vi "Example Property Node 1.vi"() -> ()   [LabVIEW 2018]
panel:
  out "Connected Wire":refnum<vi>
  out "error out":errorcluster
  out "reference out":refnum<vi>
  in  "error in (no error)":errorcluster
  in  "reference":refnum<vi>
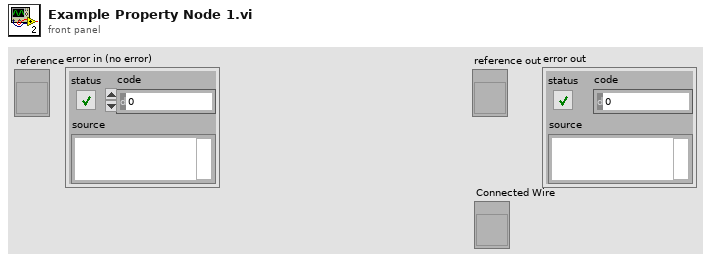
[diagram p1: front panel]
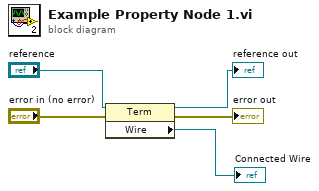
[diagram p0: block diagram]
diagram:
  n1 = property class="Term"(reference="reference", error in="error in (no error)") -> (reference out=→"reference out":refnum<vi>, error out=→"error out":errorcluster, "Wire"=→"Connected Wire":refnum<vi>)
